vi "Space Constant.vi"() -> (0 "String":string)   [LabVIEW 2024]
doc: "<p>Use this constant to supply a one-character space string to the block diagram.</p>"
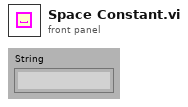
[diagram p1: front panel]
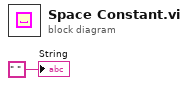
[diagram p0: block diagram]
diagram:
  "String" <- " "
